vi "SaveOrigin.vi"   [LabVIEW 2017]
uses:
  Settings/Traverse-Settings-Global.vi
types:
  T1 = typedef "Settings-Control.ctl" = cluster{"Acceleration":dbl[], "Deceleration":dbl[], "Max Velocity":dbl[], "Speed":dbl, "Pulse/Degree":dbl, "Degre Factor":dbl[], "mm/rotation":dbl[], "Traverse Name":string}
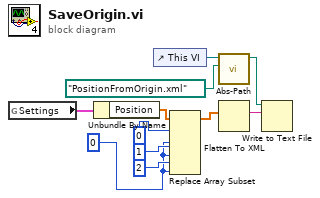
[diagram p0: block diagram]
diagram:
  w1 = 0 ("index")
  n1 = global read "Traverse-Settings-Global.vi" "Settings"() -> (w3:T1)
  n2 = Unbundle By Name(w3) -> ("Position"=w2:dbl[])
  n3 = control-ref of="This VI"() -> (w10:refnum<vi>)
  n4 = Replace Array Subset(array=w2, new element #1=w1, index #1=0 ("index"), new element #2=w1, index #2=1 ("index"), new element #3=w1, index #3=2 ("index")) -> (w4:dbl[])
  n5 = call "Abs-Path.vi"("filename"=path "PositionFromOrigin.xml" ("file (use dialog)"), "Vi in path"=w10) -> ("Full path"=w11:path)  [unwired: 9 in]
  n6 = Flatten To XML(anything=w4) -> (xml string=w9:string)
  n7 = Write to Text File(file (use dialog)=w11, text=w9) -> ()  [unwired: 2 in, 3 out]
